vi "String to Control.vi"(9 "Limit":refnum<vi>, 11 "Multicolumn Listbox":refnum<vi>) -> ()   [LabVIEW 2019, in "TestSetup.lvlib" / "TestSetup.lvclass"]
uses:
  TestSetup.lvclass
  Limit.ctl
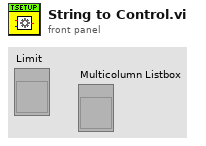
[diagram p1: front panel]
types:
  T1 = typedef "TestSetup.lvlib/TestSetup.lvclass/Limit.ctl" = cluster{"ItemName":string, "Type":enum16{"I8", "I16", "I32", "I64", "U8", "U16", "U32", "U64", "Double Float", "Boolean", "String", "Numeric Array", "String Array"}, "LowLimit":string, "HighLimit":string}
  T2 = enum16{"I8", "I16", "I32", "I64", "U8", "U16", "U32", "U64", "Double Float", "Boolean", "String", "Numeric Array", "String Array"}
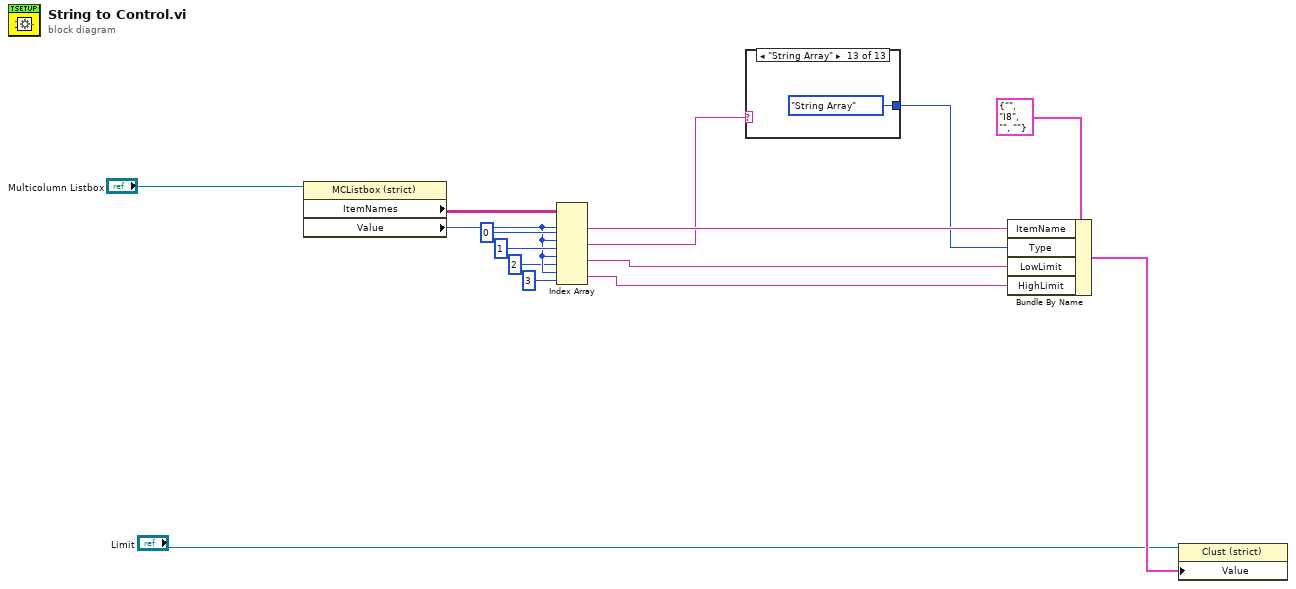
[diagram p0: block diagram]
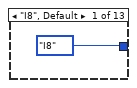
[diagram p2: hidden frame]
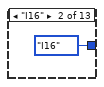
[diagram p3: hidden frame]
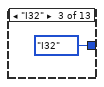
[diagram p4: hidden frame]
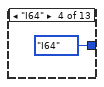
[diagram p5: hidden frame]
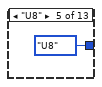
[diagram p6: hidden frame]
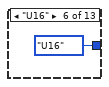
[diagram p7: hidden frame]
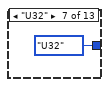
[diagram p8: hidden frame]
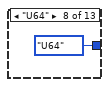
[diagram p9: hidden frame]
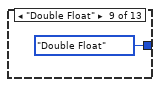
[diagram p10: hidden frame]
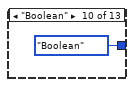
[diagram p11: hidden frame]
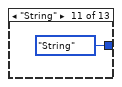
[diagram p12: hidden frame]
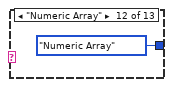
[diagram p13: hidden frame]
diagram:
  n1 = property class="MCListbox (strict)"(reference="Multicolumn Listbox") -> ("ItemNames"=w14:string[][], "Value"=w11:i32)  [unwired: 1 in, 2 out]
  n2 = Index Array(array=w14, index (row) #1=w11, index (col) #1=0 ("disabled index (col)"), index (row) #2=w11, index (col) #2=1 ("disabled index (col)"), index (row) #3=w11, index (col) #3=2 ("disabled index (col)"), index (row) #4=w11, index (col) #4=3 ("disabled index (col)")) -> (element #1=w6:string, element #2=w3:string, element #3=w5:string, element #4=w4:string)
  n3 = case shown="\"String Array\"" w3 {
    tunnel: [T2."I8" ("Type") T2."I16" ("Type") T2."I32" ("Type") T2."I64" ("Type") T2."U8" ("Type") T2."U16" ("Type") T2."U32" ("Type") T2."U64" ("Type") T2."Double Float" ("Type") T2."Boolean" ("Type") T2."String" ("Type") T2."Numeric Array" ("Type") T2."String Array" ("Type")] -> w1
    frame "I8", Default {
    }
    frame "I16" {
    }
    frame "I32" {
    }
    frame "I64" {
    }
    frame "U8" {
    }
    frame "U16" {
    }
    frame "U32" {
    }
    frame "U64" {
    }
    frame "Double Float" {
    }
    frame "Boolean" {
    }
    frame "String" {
    }
    frame "Numeric Array" {
    }
    frame "String Array" {
    }
  }
  n4 = Bundle By Name(cluster=T1 {"ItemName"="", "Type"=enum."I8", "LowLimit"="", "HighLimit"=""} ("Value"), "ItemName"=w6, "Type"=w1, "LowLimit"=w5, "HighLimit"=w4) -> (w7:T1)
  n5 = property class="Clust (strict)"(reference="Limit", "Value"=w7) -> ()  [unwired: 1 in, 2 out]
